vi "Mathcad Save large Arrays.vi"(8 "error in (no error)":errorcluster, 11 "file text":string) -> (0 "error out":errorcluster, 3 "file text w save large arrays":string)   [LabVIEW 2012]
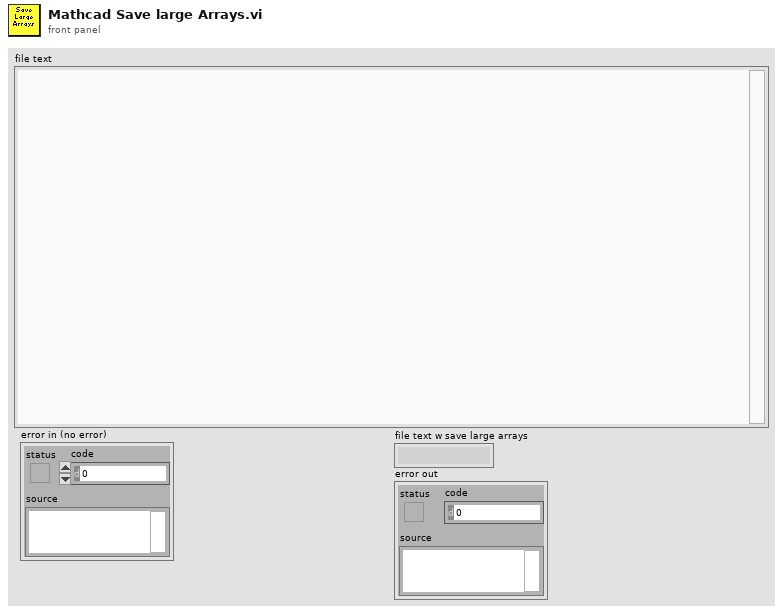
[diagram p1: front panel]
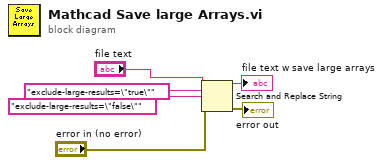
[diagram p0: block diagram]
diagram:
  n1 = Search and Replace String(input string="file text", search string="exclude-large-results=\"true\"" ("regular expression"), replace string="exclude-large-results=\"false\"" ("replace string (\"\")"), error in="error in (no error)") -> (result string=→"file text w save large arrays":string, error out=→"error out":errorcluster)  [unwired: 4 in, 2 out]
